vi "emptyProcess.vi"(8 "error in (no error)":errorcluster, 11 "ID":i32=1336) -> (0 "error out":errorcluster, 1 "ProcessWorkingSetSize min":i32=204800, 2 "ProcessWorkingSetSize max":i32=1413120, 6 "return":i32=87)   [LabVIEW 2020]
uses:
  processHandles.dll
panel:
  in  "min":i32
  in  "max":i32
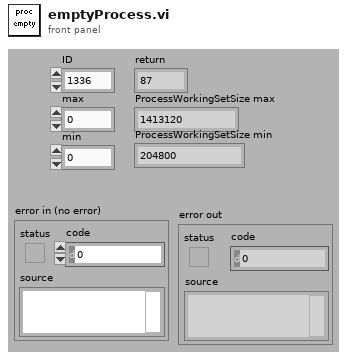
[diagram p1: front panel]
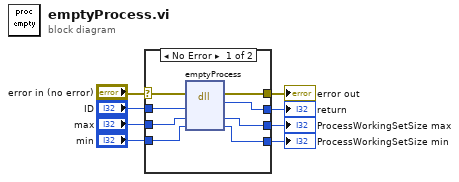
[diagram p0: block diagram]
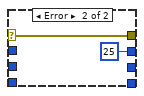
[diagram p2: hidden frame]
diagram:
  n1 = case shown="No Error" "error in (no error)" {
    selector: "error in (no error)" -> [w9 w18]
    tunnel: "ID" -> [w16 _]
    tunnel: "max" -> [w15 _]
    tunnel: "min" -> [w14 _]
    tunnel: [w13 _] -> w5
    tunnel: [w12 _] -> w4
    tunnel: [w11 25 ("return type")] -> w3
    tunnel: [w10 w18] -> w2
    frame No Error {
      n2 = dll-call lib="E:/LabVIEW 2020 Toolkits/toolkits_lv2020_32bit/TaskManager/processHandles.dll" fn="emptyProcess"(error in=w9, "ID"=w16, "max"=w15, "min"=w14) -> (error out=w10:errorcluster, "return type"=w11:i32, "max"=w13:i32, "min"=w12:i32)  [unwired: 3 in, 1 out]
    }
    frame Error {
    }
  }
  "return" <- w3
  "ProcessWorkingSetSize max" <- w5
  "ProcessWorkingSetSize min" <- w4
  "error out" <- w2
